vi "Flush Idle.vi"(8 "error in (no error)":errorcluster, 10 "State":string, 11 "Queue in":refnum<queue>) -> (0 "error out":errorcluster, 3 "Queue out":refnum<queue>)   [LabVIEW 2016]
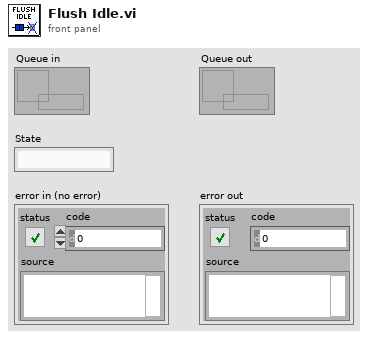
[diagram p1: front panel]
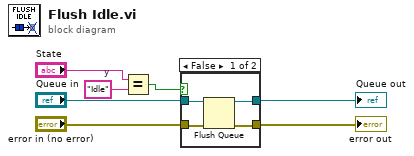
[diagram p0: block diagram]
diagram:
  w6 = "Idle"  # y
  n1 = Equal?(x="State", y=w6) -> (x = y?=w7:bool)
  n2 = case shown="False" w7 {
    tunnel: "Queue in" -> [w11 w13]
    tunnel: [w9 w13] -> w2
    tunnel: [w8 w12] -> w3
    tunnel: "error in (no error)" -> [w10 w12]
    frame False {
      n3 = Flush Queue(queue=w11, error in (no error)=w10) -> (queue out=w9:refnum<queue>, error out=w8:errorcluster)  [unwired: 1 out]
    }
    frame True {
    }
  }
  "error out" <- w3
  "Queue out" <- w2
